vi "Insert Conditional.vi"(0 "Test Executive in":refnum<class "Test Executive.lvclass">, 1 "Name":string, 2 "Unique ID":string, 3 "Insertion Index":i32=-1, 4 "Assertion":refnum<class "Assert.lvclass">, 5 "error in (no error)":errorcluster, 6 "Parent ID":string, 7 "Variable X":string, 9 "Variable Y":string, 11 "Passing Executive":string, 13 "Failing Executive":string) -> (12 "Unique ID out":string, 14 "Test Executive out":refnum<class "Test Executive.lvclass">, 17 "Replaced?":bool, 19 "error out":errorcluster)   [LabVIEW 2020, in "Test Executive.lvlib" / "Test Executive.lvclass"]
uses:
  <vilib>/gpm_packages/@cs/test-executive/Source/Test Executive/TestExecutive/Test Executive.lvclass
  <vilib>/gpm_packages/@cs/run-time-assertions/Source/Assert/Assert.lvclass
  <vilib>/gpm_packages/@cs/test-executive/Source/Test Executive/Conditional/Conditional.lvclass
  <vilib>/gpm_packages/@cs/test-executive/Source/Test Executive/TestExecutive/Test Executive.lvclass/Test Executive.ctl
  952998c2-1566-4e65-881a-35de7e1992d2.vi
  23b94a86-9bb9-4b71-8b9c-7a2918f73b68.vi
  cd60f2f5-d17b-4d8e-a806-1ec299b54eab.vi
  6ed1b01b-abe1-4cdd-99cc-63e72e6d2583.vi
  4433f8a1-5259-4890-a279-471161dc7057.vi
  a9ffea48-b162-481b-8c80-0ee3b163fd09.vi
  e0cf0242-6218-4a1f-8dae-9a6f9690ba96.vi
  <vilib>/gpm_packages/@cs/linked-list/Source/Linked List/ILinkedList/ILinked List.lvclass
  <vilib>/gpm_packages/@cs/linked-list/Source/Linked List/Linked List Ref/Linked List Ref.lvclass
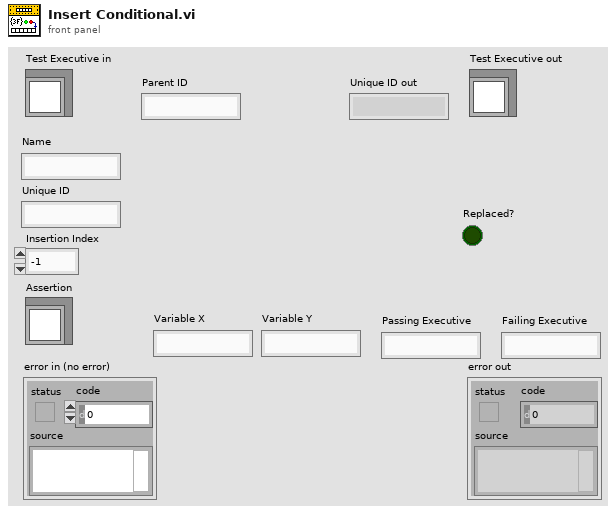
[diagram p1: front panel]
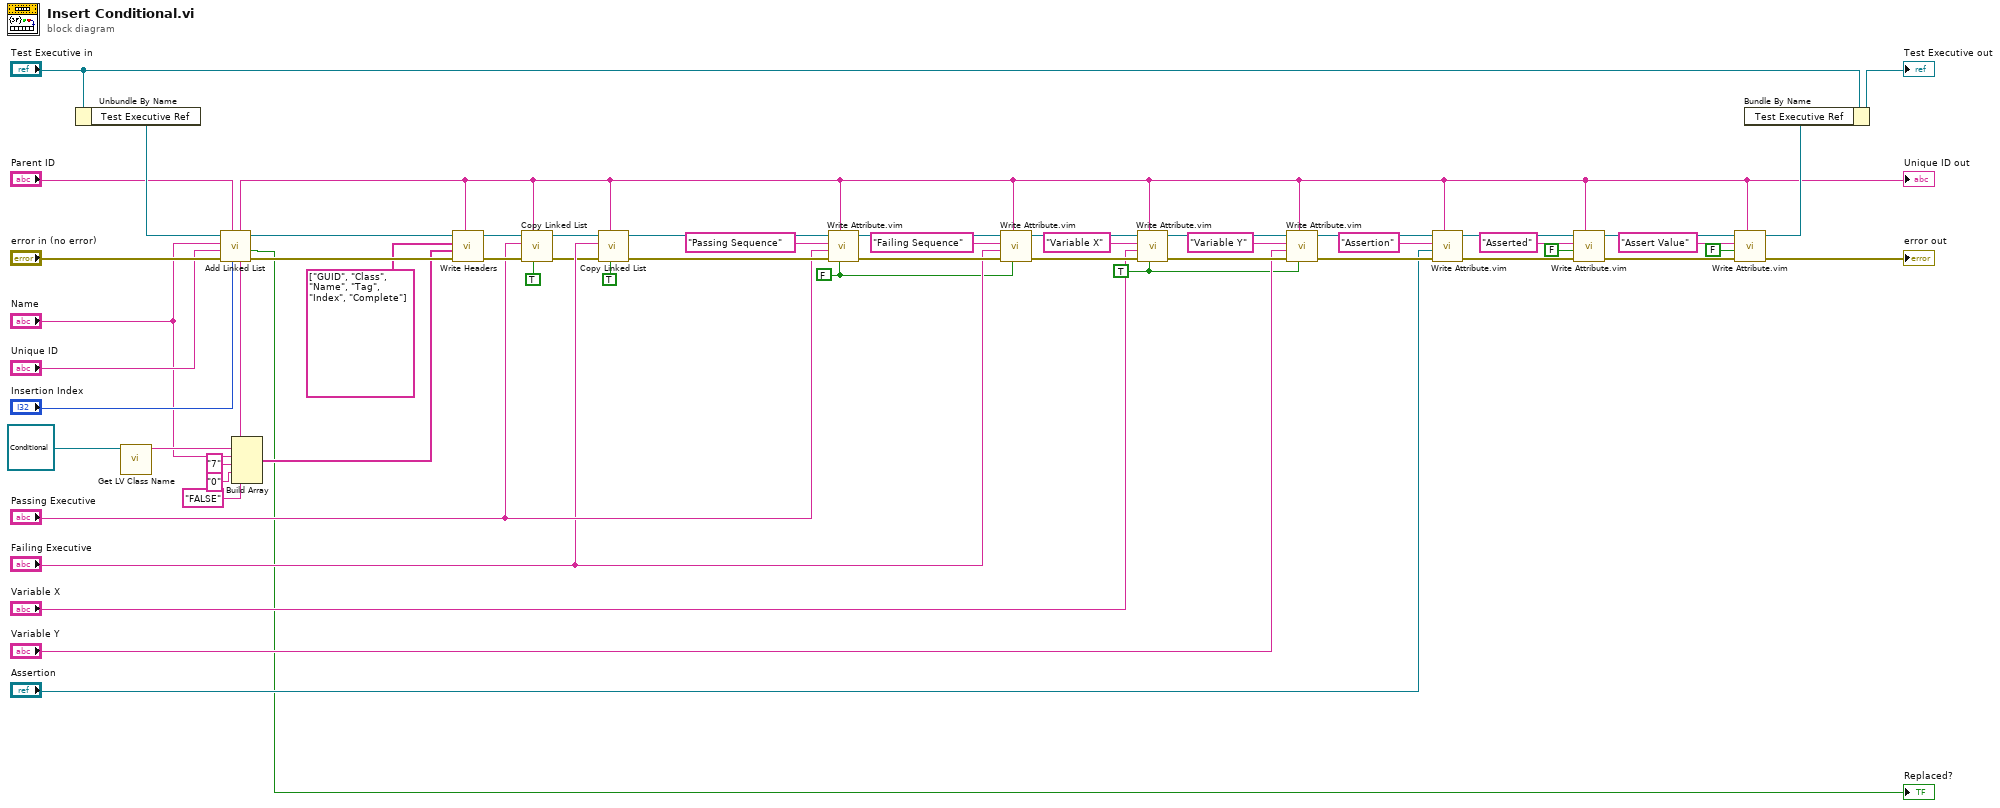
[diagram p0: block diagram]
diagram:
  w1 = FALSE ("Pointer?")
  w2 = TRUE ("Pointer?")
  n1 = Unbundle By Name("Test Executive in") -> ("Test Executive Ref"=w54:refnum<data-value>)
  n2 = call <vilib>:"Get LV Class Name.vi"("object"=refnum<class "Conditional.lvclass"> refnum ("Test Executive.lvlib:Conditional.lvclass")) -> ("class name"=w46:string)  [unwired: 9 in, 1 out]
  n3 = call <vilib>:"Add Linked List.vi"("Insertion Index"="Insertion Index", "Parent ID"="Parent ID", "error in (no error)"="error in (no error)", "Linked List ID"="Unique ID", "Name"="Name", "Linked List Ref"=w54) -> ("error out"=w50:errorcluster, "Replaced?"=→"Replaced?":bool, "Linked List Ref out"=w51:refnum<data-value>, "Linked List ID out"=w11:string)  [unwired: 2 in]
  "Unique ID out" <- w11
  n4 = Build Array(w11, w46, "Name", "7" ("element"), "0" ("element"), "FALSE" ("element")) -> (w43:string[])
  n5 = call <vilib>:"Write Headers.vi"("Linked List ID"=w11, "error in (no error)"=w50, "Header Values"=w43, "Header Names"=string[] ["GUID", "Class", "Name", "Tag", "Index", "Complete"], "Linked List Ref"=w51) -> ("error out"=w41:errorcluster, "Linked List Ref out"=w42:refnum<data-value>)  [unwired: 5 in]
  n6 = call <vilib>:"Copy Linked List.vi"("Move?"=TRUE, "New Parent Linked List ID"=w11, "error in (no error)"=w41, "Linked List ID"="Passing Executive", "Linked List Ref"=w42) -> ("error out"=w4:errorcluster, "Linked List Ref out"=w5:refnum<data-value>)  [unwired: 3 in, 2 out]
  n7 = call <vilib>:"Copy Linked List.vi"("Move?"=TRUE, "New Parent Linked List ID"=w11, "error in (no error)"=w4, "Linked List ID"="Failing Executive", "Linked List Ref"=w5) -> ("error out"=w39:errorcluster, "Linked List Ref out"=w40:refnum<data-value>)  [unwired: 3 in, 2 out]
  n8 = call "Write Attribute.vim"("Pointer?"=w1, "Linked List ID"=w11, "error in (no error)"=w39, "Attribute"="Passing Executive", "Attribute Name"="Passing Sequence", "Linked List Ref"=w40) -> ("error out"=w36:errorcluster, "Linked List Ref out"=w37:refnum<data-value>)  [unwired: 2 in, 2 out]
  n9 = call "Write Attribute.vim"("Pointer?"=w1, "Linked List ID"=w11, "error in (no error)"=w36, "Attribute"="Failing Executive", "Attribute Name"="Failing Sequence", "Linked List Ref"=w37) -> ("error out"=w32:errorcluster, "Linked List Ref out"=w34:refnum<data-value>)  [unwired: 2 in, 2 out]
  n10 = call "Write Attribute.vim"("Pointer?"=w2, "Linked List ID"=w11, "error in (no error)"=w32, "Attribute"="Variable X", "Attribute Name"="Variable X", "Linked List Ref"=w34) -> ("error out"=w29:errorcluster, "Linked List Ref out"=w30:refnum<data-value>)  [unwired: 2 in, 2 out]
  n11 = call "Write Attribute.vim"("Pointer?"=w2, "Linked List ID"=w11, "error in (no error)"=w29, "Attribute"="Variable Y", "Attribute Name"="Variable Y", "Linked List Ref"=w30) -> ("error out"=w25:errorcluster, "Linked List Ref out"=w26:refnum<data-value>)  [unwired: 2 in, 2 out]
  n12 = call "Write Attribute.vim"("Linked List ID"=w11, "error in (no error)"=w25, "Attribute"="Assertion", "Attribute Name"="Assertion", "Linked List Ref"=w26) -> ("error out"=w21:errorcluster, "Linked List Ref out"=w22:refnum<data-value>)  [unwired: 3 in, 2 out]
  n13 = call "Write Attribute.vim"("Linked List ID"=w11, "error in (no error)"=w21, "Attribute"=FALSE, "Attribute Name"="Asserted", "Linked List Ref"=w22) -> ("error out"=w16:errorcluster, "Linked List Ref out"=w17:refnum<data-value>)  [unwired: 3 in, 2 out]
  n14 = call "Write Attribute.vim"("Linked List ID"=w11, "error in (no error)"=w16, "Attribute"=FALSE, "Attribute Name"="Assert Value", "Linked List Ref"=w17) -> ("error out"=→"error out":errorcluster, "Linked List Ref out"=w13:refnum<data-value>)  [unwired: 3 in, 2 out]
  n15 = Bundle By Name(cluster="Test Executive in", "Test Executive Ref"=w13) -> (→"Test Executive out":refnum<class "Test Executive.lvclass">)
